vi "MNK_TC_to_DSC.vi"(0 "description, string":refnum<k21>="ni.var.psp://housesoftheholy/MNK_18T/MNK_TC_description", 1 "dbl var":refnum<k21>[](array[refnum])=["ni.var.psp://housesoftheholy/MNK_18T/MNK_TC_R0", "ni.var.psp://housesoftheholy/MNK_18T/MNK_TC_R1", "ni.var.psp://housesoftheholy/MNK_18T/MNK_TC_R2", "ni.var.psp://housesoftheholy/MNK_18T/MNK_TC_R3", "ni.var.psp://housesoftheholy/MNK_18T/MNK_TC_R4", "ni.var.psp://housesoftheholy/MNK_18T/MNK_TC_R5", "ni.var.psp://housesoftheholy/MNK_18T/MNK_TC_R6", "ni.var.psp://housesoftheholy/MNK_18T/MNK_TC_R7", "ni.var.psp://housesoftheholy/MNK_18T/MNK_TC_T0", "ni.var.psp://housesoftheholy/MNK_18T/MNK_TC_T1", "ni.var.psp://housesoftheholy/MNK_18T/MNK_TC_T2", "ni.var.psp://housesoftheholy/MNK_18T/MNK_TC_T3", "ni.var.psp://housesoftheholy/MNK_18T/MNK_TC_T4", "ni.var.psp://housesoftheholy/MNK_18T/MNK_TC_T5", "ni.var.psp://housesoftheholy/MNK_18T/MNK_TC_T6", "ni.var.psp://housesoftheholy/MNK_18T/MNK_TC_T7", "ni.var.psp://housesoftheholy/MNK_18T/MNK_TC_I0", "ni.var.psp://housesoftheholy/MNK_18T/MNK_TC_I1", "ni.var.psp://housesoftheholy/MNK_18T/MNK_TC_I2", "ni.var.psp://housesoftheholy/MNK_18T/MNK_TC_I3", "", "", "", "", ""], 2 "dbl":dbl[](array[numeric]), 5 "String In":string, 7 "calibration string":refnum<k21>="ni.var.psp://housesoftheholy/MNK_18T/MNK_TC_calibration", 9 "String In 2":string, 11 "error in (no error)":errorcluster) -> (15 "error out":errorcluster)   [LabVIEW 2013]
panel:
  # "MNK TC to DSC"
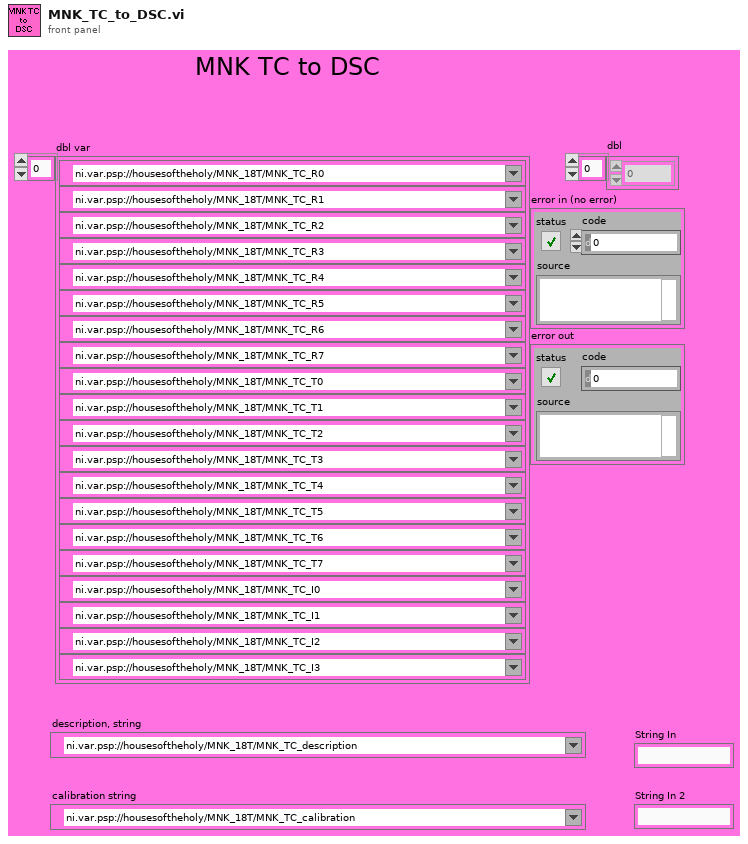
[diagram p1: front panel]
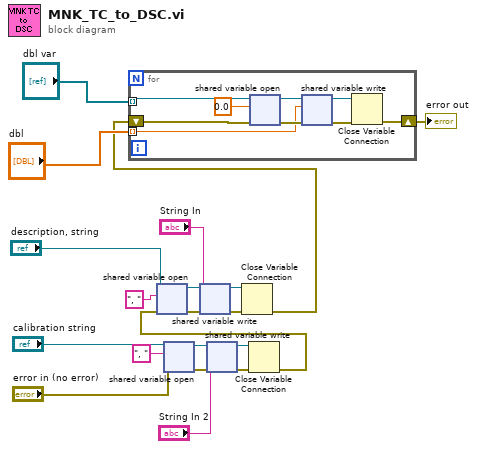
[diagram p0: block diagram]
diagram:
  n1 = shared-variable-open("calibration string", "error in (no error)", ", " ("string")) -> (w17:refnum<k21>, w16:errorcluster)  [unwired: 1 in]
  n2 = shared-variable-write(w17, w16, "String In 2") -> (w18:refnum<k21>, w15:errorcluster)
  n3 = Close Variable Connection(8:w15, 11:w18) -> (0:w4:errorcluster)
  n4 = shared-variable-open("description, string", w4, ", " ("string")) -> (w12:refnum<k21>, w11:errorcluster)  [unwired: 1 in]
  n5 = shared-variable-write(w12, w11, "String In") -> (w13:refnum<k21>, w10:errorcluster)
  n6 = Close Variable Connection(8:w10, 11:w13) -> (0:w3:errorcluster)
  n7 = for {
    tunnel: "dbl var" -> [w24] mode=indexing
    tunnel: "dbl" -> [w23] mode=indexing
    shift-right: [w22] -> w1
    shift-left: w3 -> [w21]
    n8 = shared-variable-open(w24, w21, 0.0) -> (w27:refnum<k21>, w28:errorcluster)  [unwired: 1 in]
    n9 = shared-variable-write(w27, w28, w23) -> (w26:refnum<k21>, w29:errorcluster)
    n10 = Close Variable Connection(8:w29, 11:w26) -> (0:w22:errorcluster)
  }
  "error out" <- w1
